vi "miles to meters.vi"() -> ()   [LabVIEW 2019]
panel:
  in  "Tab Control":enum32{"Conversion"}(tab)
  out "Meters":dbl
  in  "stop":bool
  out "Miles":dbl
  in  "Feet":i32
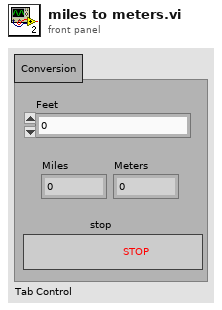
[diagram p1: front panel]
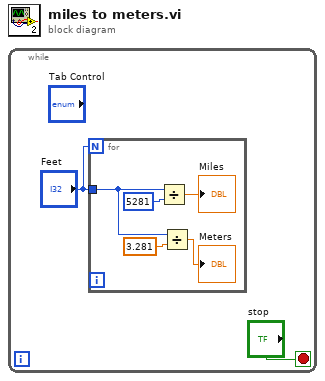
[diagram p0: block diagram]
diagram:
  n1 = while {
    stop <- "stop" stop-if-true
    n2 = for {
      N: "Feet" -> [_]
      tunnel: "Feet" -> [w4]
      n3 = Divide(x=w4, y=5281) -> (x/y=→"Miles":dbl)
      n4 = Divide(x=w4, y=3.281) -> (x/y=→"Meters":dbl)
    }
  }
